vi "Write Configuration Class Name.vi"(8 "error in (no error)":errorcluster, 10 "Configuration Class Name":string[](array[string]), 11 "Targets in":refnum<class "Targets.lvclass">) -> (0 "error out":errorcluster, 3 "Targets out":refnum<class "Targets.lvclass">)   [LabVIEW 2013, in "PL Framework Configuration Tool.lvlib" / "Targets.lvclass"]
uses:
  Targets.lvclass
  Targets.lvclass/Targets.ctl
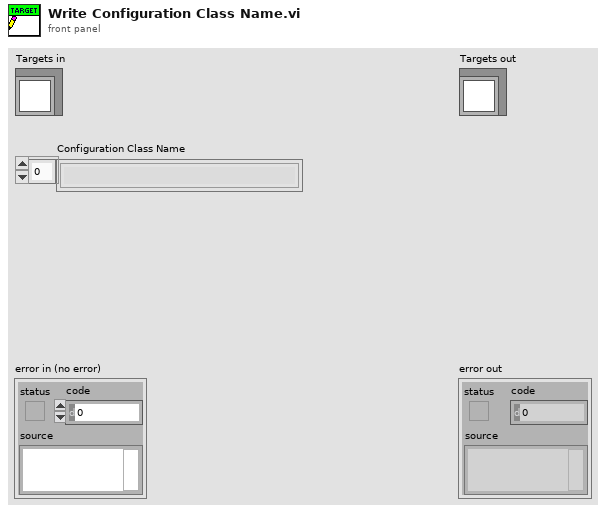
[diagram p1: front panel]
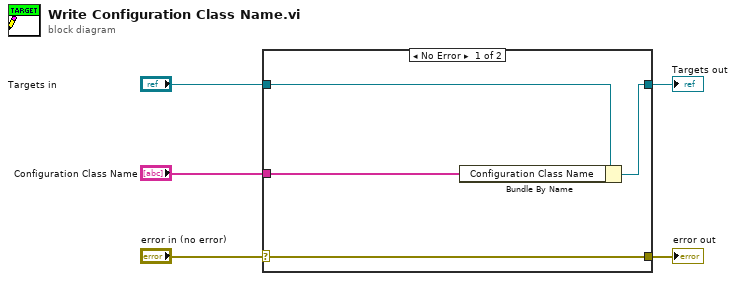
[diagram p0: block diagram]
diagram:
  n1 = case shown="No Error" "error in (no error)" {
    selector: "error in (no error)" -> [w9 w10]
    tunnel: [w9 w10] -> w4
    tunnel: [w7 w11] -> w2
    tunnel: "Targets in" -> [w8 w11]
    tunnel: "Configuration Class Name" -> [w6 _]
    frame No Error {
      n2 = Bundle By Name(cluster=w8, "Configuration Class Name"=w6) -> (w7:refnum<class "Targets.lvclass">)
    }
    frame Error {
    }
  }
  "error out" <- w4
  "Targets out" <- w2
